vi "prompt.vi"(0 "connection ID":refnum<k5>, 1 "type":string, 5 "JSON Tree In (JSON Object)":variant, 7 "default value":string, 9 "timeout ms":i32=10000, 11 "error in":errorcluster, 12 "Display Style":u32) -> (4 "connection ID out":refnum<k5>, 6 "cancelled?":bool, 15 "error out":errorcluster)   [LabVIEW 2010]
uses:
  i3-json-1.0.0-10/JSON Parsing/Get Object Parameter Files/Get Object Parameter - Array.vi
  i3-json-1.0.0-10/JSON Parsing/Get Array Value at Index Files/Get Array Value at Index - String.vi
  i3-json-1.0.0-10/JSON Generation/Create Value Files/Create Value - Null.vi
  i3-json-1.0.0-10/JSON Generation/Create Value Files/Create Value - String.vi
  i3-json-1.0.0-10/i3-json.lvlib
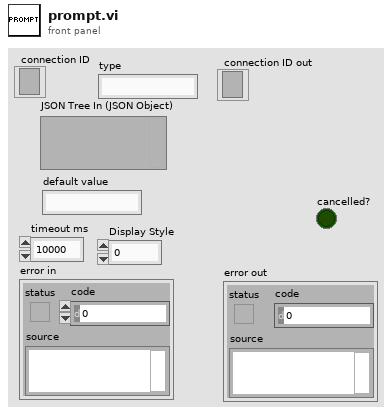
[diagram p1: front panel]
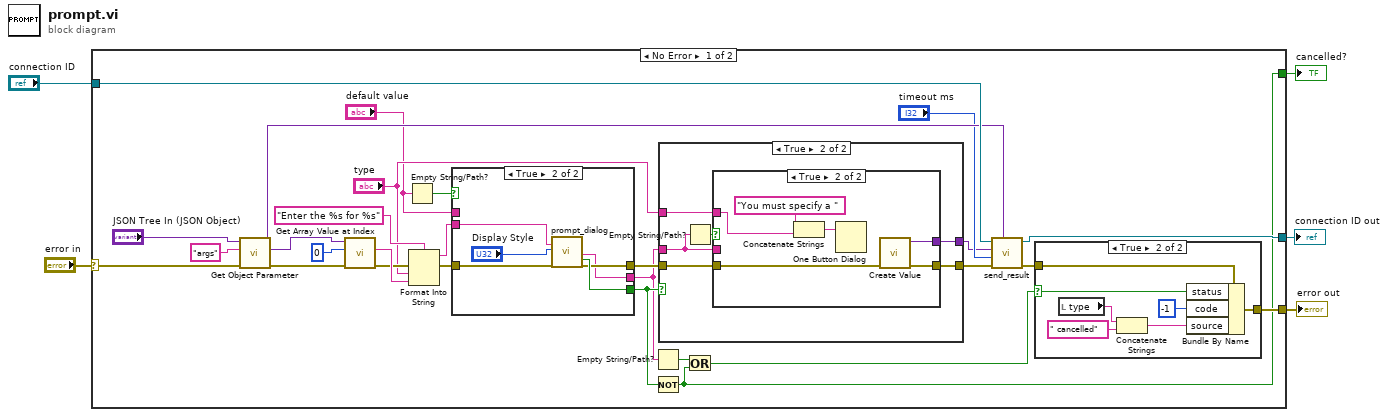
[diagram p0: block diagram]
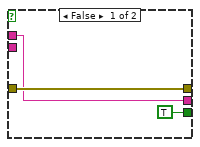
[diagram p2: hidden frame]
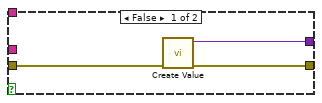
[diagram p3: hidden frame]
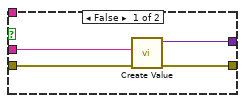
[diagram p4: hidden frame]
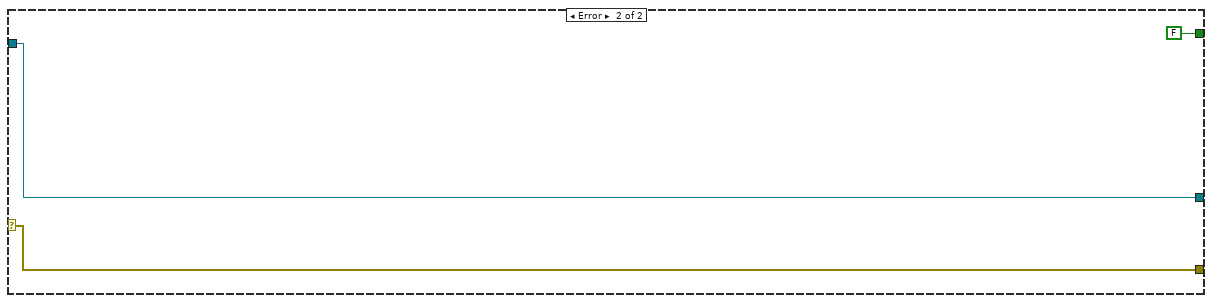
[diagram p6: hidden frame]
diagram:
  n1 = case shown="No Error" "error in" {
    selector: "error in" -> [w8 w71]
    tunnel: "connection ID" -> [w29 w72]
    tunnel: [w26 w72] -> w4
    tunnel: [w24 w71] -> w3
    tunnel: [w10 FALSE] -> w2
    frame No Error {
      n2 = call-poly "Get Object Parameter.vi"("error in (no error)"=w8, "Parameter Name"="args" ("name"), "JSON Tree In (JSON Object)"="JSON Tree In (JSON Object)") -> ("error out"=w30:errorcluster, "JSON Array"=w32:variant, "JSON Tree Out Passthrough"=w28:variant)  [unwired: 5 in, 1 out]
      n3 = call-poly "Get Array Value at Index.vi"("error in (no error)"=w30, "Index"=0, "JSON Tree In (JSON Array)"=w32) -> ("error out"=w18:errorcluster, "String Value"=w21:string)  [unwired: 5 in, 2 out]
      n4 = Empty String/Path?(string/path="default value") -> (empty?=w7:bool)
      n5 = Format Into String(format string="Enter the %s for %s", error in=w18, "type", w21) -> (resulting string=w20:string, error out=w17:errorcluster)  [unwired: 1 in]
      n6 = case shown="True" w7 {
        tunnel: w20 -> [_ w42]
        tunnel: [TRUE ("OK") w41] -> w19
        tunnel: w17 -> [w36 w40]
        tunnel: [w36 w39] -> w16
        tunnel: [w35 w38] -> w12
        tunnel: "default value" -> [w35 _]
        frame False {
        }
        frame True {
          n7 = call "prompt_dialog.vi"("caption"=w42, "Display Style"="Display Style", "error in (no error)"=w40) -> ("Value"=w38:string, "OK"=w41:bool, "error out"=w39:errorcluster)  [unwired: 14 in]
        }
      }
      n8 = Empty String/Path?(string/path=w12) -> (empty?=w11:bool)
      n9 = Not(x=w19) -> (.not. x?=w10:bool)
      n10 = case shown="True" w19 {
        tunnel: w12 -> [_ w46]
        tunnel: w16 -> [w43 w50]
        tunnel: [w44 w49] -> w15
        tunnel: [w45 w48] -> w14
        tunnel: "type" -> [_ w47]
        frame False {
          n11 = call-poly "Create Value.vi"("error in (no error)"=w43) -> ("error out"=w44:errorcluster, "JSON Tree"=w45:variant)  [unwired: 9 in]
        }
        frame True {
          n12 = Empty String/Path?(string/path=w46) -> (empty?=w51:bool)
          n13 = case shown="True" w51 {
            tunnel: w50 -> [w55 w57]
            tunnel: w46 -> [w54 _]
            tunnel: [w53 w60] -> w49
            tunnel: [w52 w61] -> w48
            tunnel: w47 -> [_ w56]
            frame False {
              n14 = call-poly "Create Value.vi"("error in (no error)"=w55, "String"=w54) -> ("error out"=w53:errorcluster, "JSON Tree"=w52:variant)  [unwired: 8 in]
            }
            frame True {
              n15 = Concatenate Strings("You must specify a " ("message"), w56) -> (w58:string)
              n16 = One Button Dialog(message=w58) -> ()  [unwired: 1 in, 1 out]
              n17 = call-poly "Create Value.vi"("error in (no error)"=w57) -> ("error out"=w60:errorcluster, "JSON Tree"=w61:variant)  [unwired: 9 in]
            }
          }
        }
      }
      n18 = Or(x=w11, y=w10) -> (x .or. y?=w9:bool)
      n19 = call "send_result.vi"("JSON Tree In (JSON Object)"=w28, "error in"=w15, "timeout ms"="timeout ms", "result"=w14, "connection ID"=w29) -> ("error out"=w27:errorcluster, "connection ID out"=w26:refnum<k5>)  [unwired: 3 in, 2 out]
      n20 = case shown="True" w9 {
        selector: w9 -> [_ w67]
        tunnel: w27 -> [w62 w69]
        tunnel: [w62 w68] -> w24
        frame False {
        }
        frame True {
          n21 = local read "type"() -> (w64:string)
          n22 = Concatenate Strings(w64, " cancelled" ("source")) -> (w63:string)
          n23 = Bundle By Name(cluster=w69, "status"=w67, "code"=-1, "source"=w63) -> (w68:errorcluster)
        }
      }
    }
    frame Error {
    }
  }
  "connection ID out" <- w4
  "error out" <- w3
  "cancelled?" <- w2
